vi "Control - Copy.vi"() -> ()   [LabVIEW 2025]
panel:
  in  "Automation":bool
  in  "ON/OFF":bool
  out "Right Most":bool
  out "Right Middle":bool
  out "Left Middle":bool
  out "Left Most":bool
  in  "Power":dbl(slide) min=0.0 max=10.0 step=1.0 scale=0.0..10.0
  in  "Left Turn":bool
  in  "Right Turn":bool
  in  "Backward":bool
  in  "Forward":bool
  # "IR Sensors"
  # "Movement Control"
  # "Power"
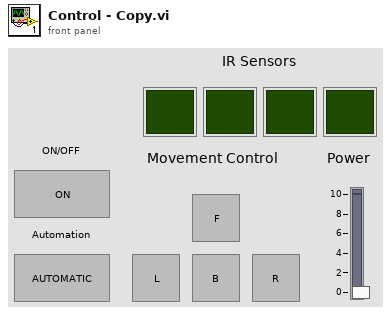
[diagram p1: front panel]
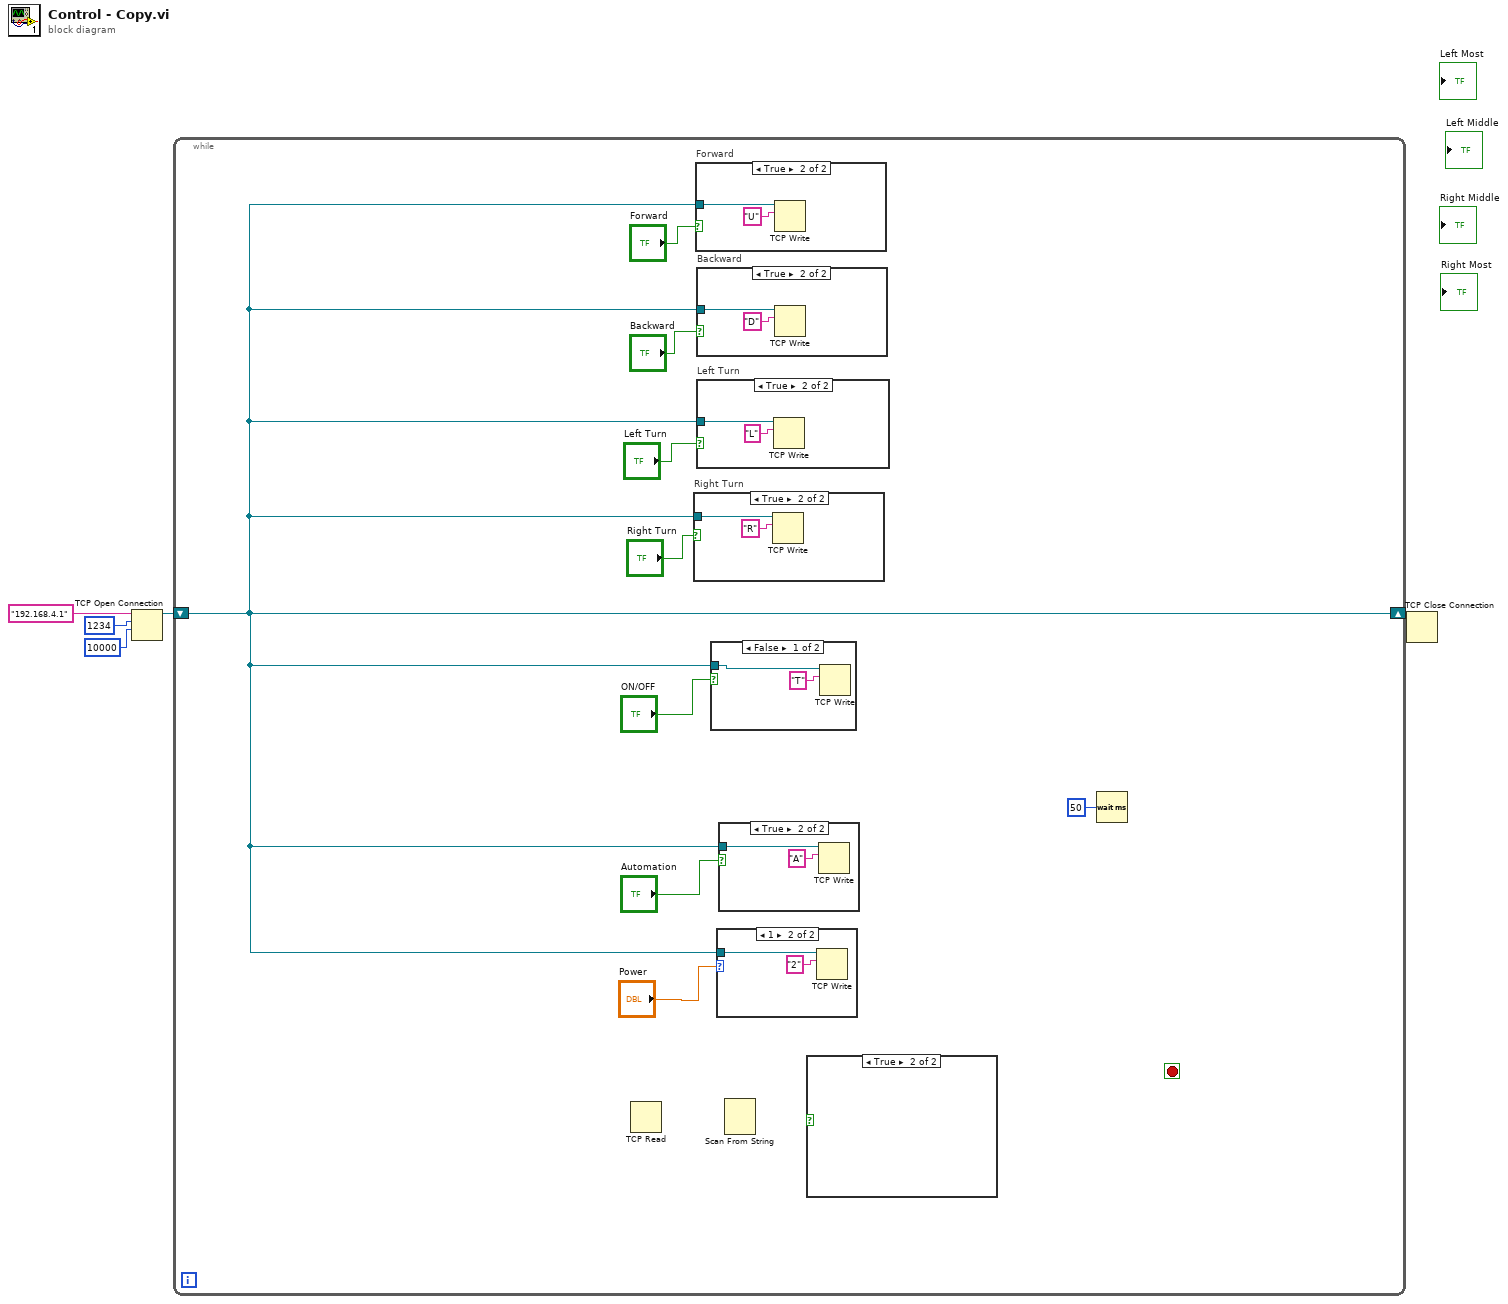
[diagram p0: block diagram]
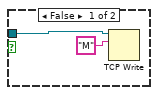
[diagram p4: hidden frame]
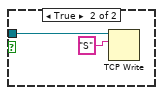
[diagram p5: hidden frame]
diagram:
  n1 = TCP Open Connection(address="192.168.4.1", remote port or service name=u16 1234, timeout ms (60000)=10000) -> (connection ID=w3:refnum<k5>)  [unwired: 2 in, 1 out]
  n2 = while {
    shift-right: [w9] -> w2
    shift-left: w3 -> [w9]
    stop <- _ stop-if-true
    n3 = TCP Read() -> ()  [unwired: 5 in, 3 out]
    n4 = case "Right Turn" shown="True" "Right Turn" {
      tunnel: w9 -> [_ w28]
      frame False {
      }
      frame True {
        n5 = TCP Write(connection ID=w28, data in="R") -> ()  [unwired: 2 in, 3 out]
      }
    }
    n6 = case "Forward" shown="True" "Forward" {
      tunnel: w9 -> [_ w32]
      frame False {
      }
      frame True {
        n7 = TCP Write(connection ID=w32, data in="U") -> ()  [unwired: 2 in, 3 out]
      }
    }
    n8 = case "Backward" shown="True" "Backward" {
      tunnel: w9 -> [_ w30]
      frame False {
      }
      frame True {
        n9 = TCP Write(connection ID=w30, data in="D") -> ()  [unwired: 2 in, 3 out]
      }
    }
    n10 = case "Left Turn" shown="True" "Left Turn" {
      tunnel: w9 -> [_ w26]
      frame False {
      }
      frame True {
        n11 = TCP Write(connection ID=w26, data in="L") -> ()  [unwired: 2 in, 3 out]
      }
    }
    n12 = case shown="False" "ON/OFF" {
      tunnel: w9 -> [w21 w24]
      frame False {
        n13 = TCP Write(connection ID=w21, data in="T") -> ()  [unwired: 2 in, 3 out]
      }
      frame True {
        n14 = TCP Write(connection ID=w24, data in="S") -> ()  [unwired: 2 in, 3 out]
      }
    }
    n15 = case shown="1" "Power" {
      tunnel: w9 -> [_ w16]
      frame 0, Default {
      }
      frame 1 {
        n16 = TCP Write(connection ID=w16, data in="2") -> ()  [unwired: 2 in, 3 out]
      }
    }
    n17 = case shown="True" "Automation" {
      tunnel: w9 -> [w17 w20]
      frame False {
        n18 = TCP Write(connection ID=w17, data in="M") -> ()  [unwired: 2 in, 3 out]
      }
      frame True {
        n19 = TCP Write(connection ID=w20, data in="A") -> ()  [unwired: 2 in, 3 out]
      }
    }
    n20 = Scan From String() -> ()  [unwired: 6 in, 3 out]
    n21 = case shown="True" {
      selector: _ -> [_ _]
      frame False {
      }
      frame True {
      }
    }
    n22 = Wait (ms)(milliseconds to wait=u32 50) -> ()  [unwired: 1 out]
  }
  n23 = TCP Close Connection(connection ID=w2) -> ()  [unwired: 2 in, 2 out]
